vi "createEvents.vi"(8 "error in (no error)":errorcluster, 11 "UserEvents in":refnum<class "UserEvents.lvclass">) -> (0 "error out":errorcluster, 3 "UserEvents out":refnum<class "UserEvents.lvclass">)   [LabVIEW 2012, in "UserEvents.lvclass"]
uses:
  UserEvents.lvclass
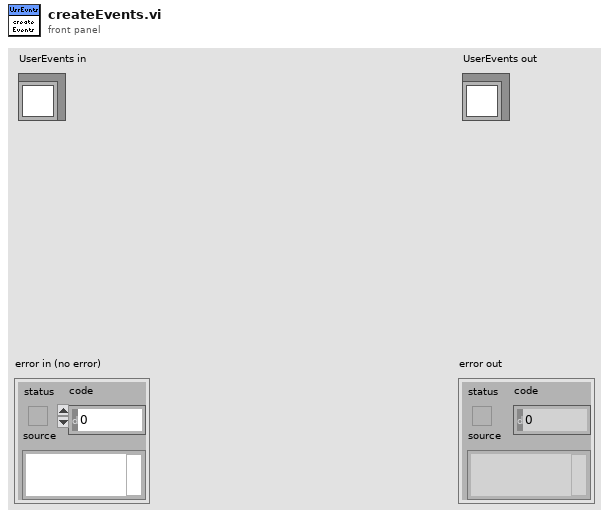
[diagram p1: front panel]
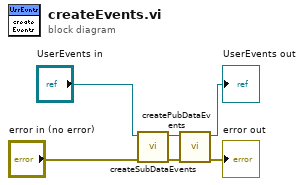
[diagram p0: block diagram]
diagram:
  n1 = call "createSubDataEvents.vi"("error in (no error)"="error in (no error)", "UserEvents in"="UserEvents in") -> ("error out"=w3:errorcluster, "UserEvents out"=w6:refnum<class "UserEvents.lvclass">)  [unwired: 8 in]
  n2 = call "createPubDataEvents.vi"("error in (no error)"=w3, "UserEvents in"=w6) -> ("error out"=→"error out":errorcluster, "UserEvents out"=→"UserEvents out":refnum<class "UserEvents.lvclass">)  [unwired: 8 in]
